vi "insert footer.vi"(6 "call chain index (1)":i32=1, 7 "vi ref (caller)":refnum<vi>, 8 "error in (no error)":errorcluster, 11 "new text (\"\")":string) -> (0 "error out":errorcluster)   [LabVIEW 2024, in "summary manager.lvlib"]
uses:
  summary manager.lvlib
  summary sections.ctl
  summary operations.ctl
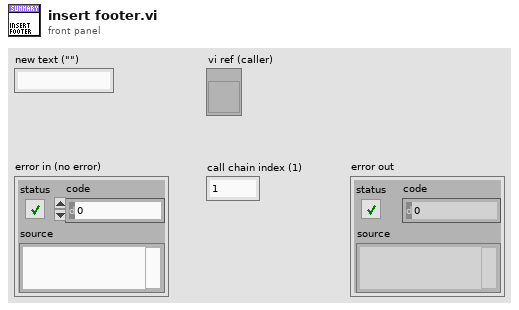
[diagram p1: front panel]
types:
  T1 = typedef "summary manager.lvlib/summary operations.ctl" = enum16{"insert", "replace", "delete"}
  T2 = typedef "summary manager.lvlib/summary sections.ctl" = enum16{"header", "body", "footer"}
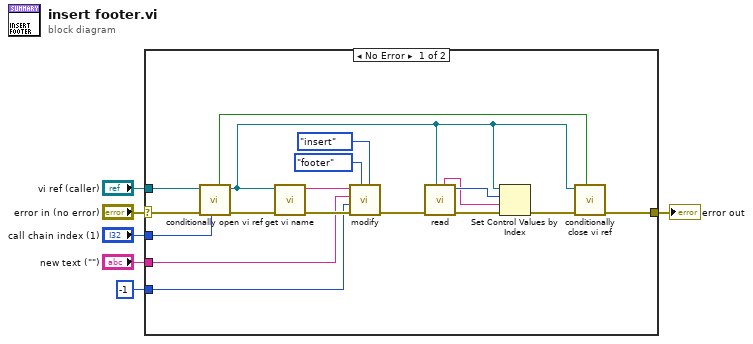
[diagram p0: block diagram]
diagram:
  n1 = case shown="No Error" "error in (no error)" {
    selector: "error in (no error)" -> [w14 w25]
    tunnel: [w13 w25] -> w5
    tunnel: "vi ref (caller)" -> [w12 _]
    tunnel: "call chain index (1)" -> [w11 _]
    tunnel: "new text (\"\")" -> [w10 _]
    tunnel: -1 -> [w9 _]
    frame No Error {
      n2 = call "conditionally open vi ref.vi"("call chain index (1)"=w11, "error in (no error)"=w14, "vi ref in"=w12) -> ("error out"=w24:errorcluster, "vi ref out"=w18:refnum<vi>, "new ref?"=w16:bool)  [unwired: 6 in]
      n3 = call "get vi name.vi"("error in (no error)"=w24, "vi ref"=w18) -> ("error out"=w23:errorcluster, "vi name"=w15:string)  [unwired: 8 in]
      n4 = call "modify.vi"("operation"=summary_operations."insert", "section"=summary_sections."footer", "error in (no error)"=w23, "index"=w9, "new text"=w10, "id"=w15) -> ("error out"=w20:errorcluster)  [unwired: 5 in]
      n5 = call "read.vi"("vi ref (caller)"=w18, "error in (no error)"=w20) -> ("error out"=w22:errorcluster, "summary control id"=w21:i32, "summary text"=w17:string)  [unwired: 4 in, 3 out]
      n6 = Set Control Values by Index(0:w18, 1:w21, 2:w17, 3:w22) -> (11:w19:errorcluster)
      n7 = call "conditionally close vi ref.vi"("new ref?"=w16, "error in (no error)"=w19, "vi ref"=w18) -> ("error out"=w13:errorcluster)  [unwired: 8 in]
    }
    frame Error {
    }
  }
  "error out" <- w5
